vi "CAPFM-Save Data.vi"(0 "Expt State":T1, 5 "CAPFM Params":T2, 11 "error in":errorcluster, 12 "Analysis":T9, 13 "Notes":string) -> (4 "Expt State Out":T1, 15 "error out":errorcluster)   [LabVIEW 2020]
uses:
  Typedefs/CAPFM-Analysis State.ctl
  Typedefs/CAPFM-All Params.ctl
  epl-vi-lib/Utility VIs/Type Defs/Left-Right ring.ctl
  Typedefs/CAPFM-Probe Params.ctl
  Typedefs/CAPFM-Masker Params.ctl
  Typedefs/CAPFM-Seq Params.ctl
  Typedefs/CAPFM-Timing Params.ctl
  Typedefs/CAPFM-Response Params.ctl
  CFTS Main Panel SubVIs/CFTS-Experiment State.ctl
  CFTS Main Panel SubVIs/CFTS-Data Type Enum.ctl
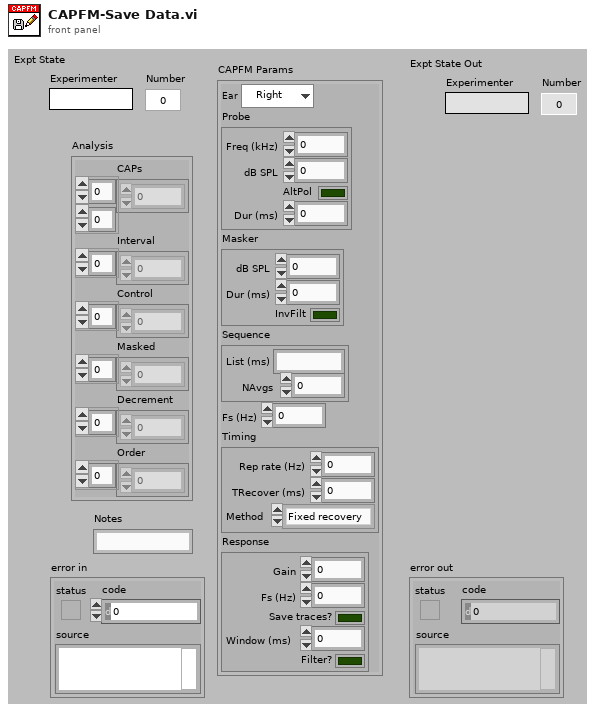
[diagram p1: front panel]
types:
  T1 = typedef "CFTS-Experiment State.ctl" = cluster{"Experimenter":string, "Number":u32, "Right":string, "Left":string, "Data Folder":path, "State File":path, "Version Info":string, "End Exposure Time":dbl, "Exposure Duration":string, "Run #":cluster{"CAP":i16, "ABR":i16, "DP":i16, "VsEP":i16, "MeasSeq":i16, "SubSeq":i16, "SFOAE":i16}}
  T2 = typedef "CAPFM-All Params.ctl" = cluster{"Ear":T3, "Probe":T4, "Masker":T5, "Sequence":T6, "Fs (Hz)":dbl, "Timing":T7, "Response":T8}
  T3 = typedef "Left-Right ring.ctl" = enum16{"Right", "Left"}
  T4 = typedef "CAPFM-Probe Params.ctl" = cluster{"Freq (kHz)":dbl, "dB SPL":dbl, "AltPol":bool, "Dur (ms)":dbl}
  T5 = typedef "CAPFM-Masker Params.ctl" = cluster{"dB SPL":dbl, "Dur (ms)":dbl, "InvFilt":bool}
  T6 = typedef "CAPFM-Seq Params.ctl" = cluster{"List (ms)":string, "NAvgs":i32}
  T7 = typedef "CAPFM-Timing Params.ctl" = cluster{"Rep rate (Hz)":dbl, "TRecover (ms)":dbl, "Method":enum16{"Fixed recovery", "Fixed rep rate"}}
  T8 = typedef "CAPFM-Response Params.ctl" = cluster{"Gain":dbl, "Fs (Hz)":dbl, "Save traces?":bool, "Window (ms)":dbl, "Filter?":bool}
  T9 = typedef "CAPFM-Analysis State.ctl" = cluster{"CAPs":dbl[][], "Interval":dbl[], "Control":dbl[], "Masked":dbl[], "Decrement":dbl[], "Order":i32[]}
  T10 = typedef "CFTS-Data Type Enum.ctl" = enum16{"CAP", "ABR", "DP", "VsEP", "MeasSeq", "SFOAE"}
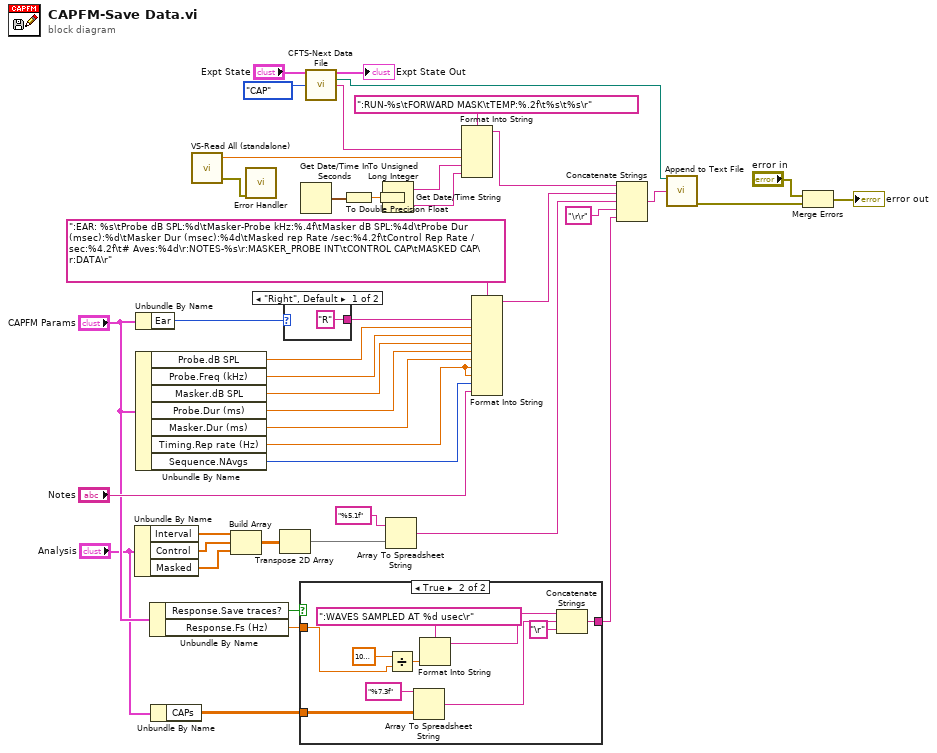
[diagram p0: block diagram]
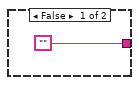
[diagram p2: hidden frame]
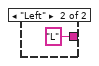
[diagram p3: hidden frame]
diagram:
  n1 = Unbundle By Name("Analysis") -> ("Interval"=w16:dbl[], "Control"=w15:dbl[], "Masked"=w14:dbl[])
  n2 = Unbundle By Name("CAPFM Params") -> ("Ear"=w34:T3)
  n3 = Unbundle By Name("CAPFM Params") -> ("Probe.dB SPL"=w31:dbl, "Probe.Freq (kHz)"=w30:dbl, "Masker.dB SPL"=w29:dbl, "Probe.Dur (ms)"=w28:dbl, "Masker.Dur (ms)"=w27:dbl, "Timing.Rep rate (Hz)"=w26:dbl, "Sequence.NAvgs"=w25:i32)
  n4 = Unbundle By Name("CAPFM Params") -> ("Response.Save traces?"=w7:bool, "Response.Fs (Hz)"=w6:dbl)
  n5 = Unbundle By Name("Analysis") -> ("CAPs"=w3:dbl[][])
  n6 = call "VS-Read All (standalone).vi"() -> ("error out"=w1:errorcluster, "Temperature (C)"=w2:dbl)  [unwired: 3 in, 1 out]
  n7 = Build Array(w16, w15, w14) -> (w13:dbl[][])
  n8 = call "Error Handler.vi"("error in (no error)"=w1) -> ()  [unwired: 13 in, 2 out]
  n9 = Transpose 2D Array(2D array=w13) -> (transposed array=w11:dbl[][])
  n10 = case shown="\"Right\", Default" w34 {
    tunnel: ["R" "L"] -> w33
    frame "Right", Default {
    }
    frame "Left" {
    }
  }
  n11 = case shown="True" w7 {
    tunnel: w6 -> [_ w55]
    tunnel: ["" w53] -> w5
    tunnel: w3 -> [_ w50]
    frame False {
    }
    frame True {
      n12 = Divide(x=1000000.0, y=w55) -> (x/y=w54:dbl)
      n13 = Array To Spreadsheet String(array=w50, 3:"%7.3f") -> (spreadsheet string=w49:string)  [unwired: 1 in]
      n14 = Format Into String(format string=":WAVES SAMPLED AT %d usec\r", w54) -> (resulting string=w52:string)  [unwired: 2 in, 1 out]
      n15 = Concatenate Strings(w52, w49, "\r" ("string")) -> (w53:string)
    }
  }
  n16 = Get Date/Time In Seconds() -> (seconds since 1Jan1904=w37:timestamp)
  n17 = call "CFTS-Next Data File.vi"("Expt State"="Expt State", "Data Type"=CFTS-Data_Type_Enum."CAP") -> ("Expt State out"=→"Expt State Out":T1, "Datafile path"=w17:path, "run #"=w40:string)  [unwired: 9 in, 2 out]
  n18 = To Double Precision Float(number=w37) -> (double precision float=w38:dbl)
  n19 = To Unsigned Long Integer(number=w38) -> (unsigned 32bit integer=w39:u32)
  n20 = Get Date/Time String(seconds (now)=w39) -> (date string=w36:string, time string=w35:string)  [unwired: 2 in]
  n21 = Array To Spreadsheet String(array=w11, 3:"%5.1f") -> (spreadsheet string=w10:string)  [unwired: 1 in]
  n22 = Format Into String(format string=":RUN-%s\tFORWARD MASK\tTEMP:%.2f\t%s\t%s\r", w40, w2, w36, w35) -> (resulting string=w19:string)  [unwired: 2 in, 1 out]
  n23 = Format Into String(format string=":EAR: %s\tProbe dB SPL:%d\tMasker-Probe kHz:%.4f\tMasker dB SPL:%4d\tProbe Dur (msec):%d\tMasker Dur (msec):%4d\tMasked rep Rate /sec:%4.2f\tControl Rep Rate /sec:%4.2f\t# Aves:%4d\r:NOTES-%s\r:MASKER_PROBE INT\tCONTROL CAP\tMASKED CAP\r:DATA\r", w33, w31, w30, w29, w28, w27, w26, w26, w25, "Notes") -> (resulting string=w18:string)  [unwired: 2 in, 1 out]
  n24 = Concatenate Strings(w19, w18, w10, "\r\r" ("string"), w5) -> (w22:string)
  n25 = call "Append to Text File.vi"("file path"=w17, "text"=w22) -> ("error out"=w23:errorcluster)  [unwired: 12 in, 1 out]
  n26 = Merge Errors("error in", w23) -> (→"error out":errorcluster)
